vi "Log Results.vi"(8 "Error In":errorcluster, 10 "Warnings":string[](array[string]), 11 "Revert Worker Config":T1={"Job Queue"=refnum, "Job Done Queue"=refnum, "Source Directory"=path "", "Unzip Directory"=path "", "Backsave Directory"=path "", "Output Directory"=path "", "Source File Name"="", "Output Path"="", "LabVIEW Version"=enum."13.0", "Archive Directory"=path ""}) -> (0 "Error Out":errorcluster, 3 "Revert Worker Config":T1={"Job Queue"=refnum, "Job Done Queue"=refnum, "Source Directory"=path "", "Unzip Directory"=path "", "Backsave Directory"=path "", "Output Directory"=path "", "Source File Name"="", "Output Path"="", "LabVIEW Version"=enum."13.0", "Archive Directory"=path ""})   [LabVIEW 2013, in "LVH-Revert.lvlib"]
uses:
  <vilib>/LabVIEW Hacker/Revert/LVH-Revert.lvlib
  <vilib>/LabVIEW Hacker/Revert/Private/Revert Worker Config.ctl
  <vilib>/National Instruments/NI Amazon Web Services (AWS) Toolkit for LabVIEW/SQS/VI Source/AWS SQS Class/AWS_SQS.lvclass
  <vilib>/National Instruments/NI Amazon Web Services (AWS) Toolkit for LabVIEW/AWS Core Lib/VI Source/Canonicals/AWS_Core Canonical Credentials/Canonical Credentials.lvclass
  <vilib>/National Instruments/NI Amazon Web Services (AWS) Toolkit for LabVIEW/AWS Core Lib/VI Source/Canonicals/AWS_Core Canonical Required Parameters/Canonical Required Parameters.lvclass
  <vilib>/National Instruments/NI Amazon Web Services (AWS) Toolkit for LabVIEW/SQS/VI Source/Canonicals/Canonical CreateQueue/Canonical CreateQueue.lvclass
  <vilib>/National Instruments/NI Amazon Web Services (AWS) Toolkit for LabVIEW/SQS/VI Source/Canonicals/Canonical ListQueues/Canonical ListQueues.lvclass
  <vilib>/National Instruments/NI Amazon Web Services (AWS) Toolkit for LabVIEW/SQS/VI Source/Canonicals/Canonical AddPermission/Canonical AddPermission.lvclass
  <vilib>/National Instruments/NI Amazon Web Services (AWS) Toolkit for LabVIEW/SQS/VI Source/Canonicals/Canonical ChangeMessageVisibility/Canonical ChangeMessageVisibility.lvclass
  <vilib>/National Instruments/NI Amazon Web Services (AWS) Toolkit for LabVIEW/SQS/VI Source/Canonicals/Canonical ChangeMessageVisibilityBatch/Canonical ChangeMessageVisibilityBatch.lvclass
  <vilib>/National Instruments/NI Amazon Web Services (AWS) Toolkit for LabVIEW/SQS/VI Source/Canonicals/Canonical DeleteMessage/Canonical DeleteMessage.lvclass
  <vilib>/National Instruments/NI Amazon Web Services (AWS) Toolkit for LabVIEW/SQS/VI Source/Canonicals/Canonical DeleteMessageBatch/Canonical DeleteMessageBatch.lvclass
  <vilib>/National Instruments/NI Amazon Web Services (AWS) Toolkit for LabVIEW/SQS/VI Source/Canonicals/Canonical GetQueueAttributes/Canonical GetQueueAttributes.lvclass
  <vilib>/National Instruments/NI Amazon Web Services (AWS) Toolkit for LabVIEW/SQS/VI Source/Canonicals/Canonical GetQueueUrl/Canonical GetQueueUrl.lvclass
  <vilib>/National Instruments/NI Amazon Web Services (AWS) Toolkit for LabVIEW/SQS/VI Source/Canonicals/Canonical ReceiveMessage/Canonical ReceiveMessage.lvclass
  <vilib>/National Instruments/NI Amazon Web Services (AWS) Toolkit for LabVIEW/SQS/VI Source/Canonicals/Canonical RemovePermission/Canonical RemovePermission.lvclass
  <vilib>/National Instruments/NI Amazon Web Services (AWS) Toolkit for LabVIEW/SQS/VI Source/Canonicals/Canonical SendMessage/Canonical SendMessage.lvclass
  <vilib>/National Instruments/NI Amazon Web Services (AWS) Toolkit for LabVIEW/SQS/VI Source/Canonicals/Canonical SendMessageBatch/Canonical SendMessageBatch.lvclass
  <vilib>/National Instruments/NI Amazon Web Services (AWS) Toolkit for LabVIEW/SQS/VI Source/Canonicals/Canonical SetQueueAttributes/Canonical SetQueueAttributes.lvclass
  <vilib>/LabVIEW Hacker/LVH-Toolbox/Common/Private/Type Defs/LabVIEW Version.ctl
  <vilib>/LabVIEW Hacker/LVH-Toolbox/Common/LVH-Common.lvlib
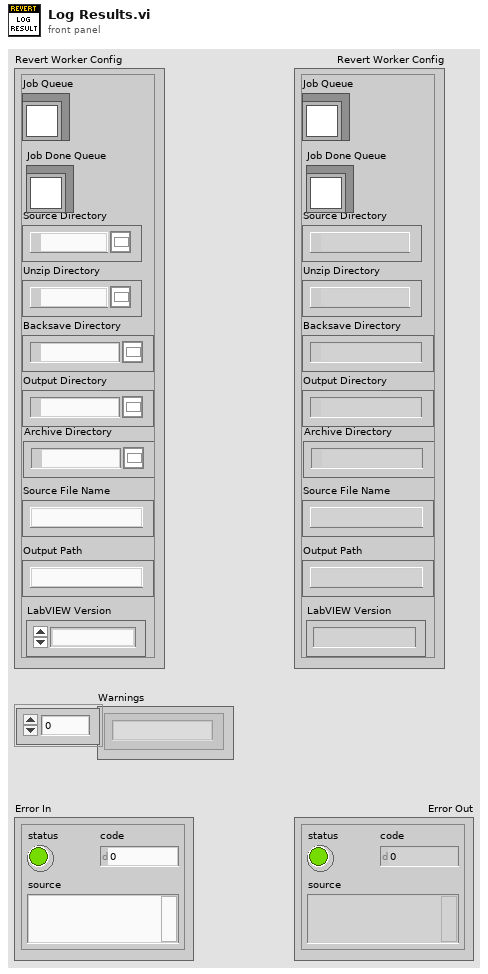
[diagram p1: front panel]
types:
  T1 = typedef "LVH-Revert.lvlib/Revert Worker Config.ctl" = cluster{"Job Queue":refnum<class "AWS_SQS.lvclass">, "Job Done Queue":refnum<class "AWS_SQS.lvclass">, "Source Directory":path, "Unzip Directory":path, "Backsave Directory":path, "Output Directory":path, "Source File Name":string, "Output Path":string, "LabVIEW Version":T2, "Archive Directory":path}
  T2 = typedef "LVH-Toolbox.lvlib/LVH-Common.lvlib/LabVIEW Version.ctl" = enum16{"8.0", "8.2", "8.6", "9.0", "10.0", "11.0", "12.0", "13.0"}
  T3 = enum16{"open", "replace", "create", "open or create", "replace or create", "replace or create with confirmation"}
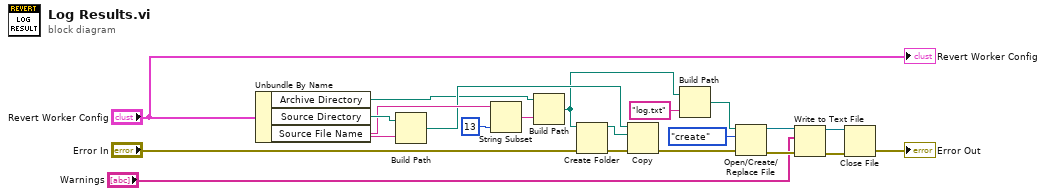
[diagram p0: block diagram]
diagram:
  n1 = Unbundle By Name("Revert Worker Config") -> ("Archive Directory"=w1:path, "Source Directory"=w7:path, "Source File Name"=w6:string)
  n2 = Build Path(base path=w7, name or relative path=w6) -> (appended path=w5:path)
  n3 = String Subset(string=w6, length (rest)=13 ("length (rest)")) -> (substring=w20:string)  [unwired: 1 in]
  n4 = Build Path(base path=w1, name or relative path=w20) -> (appended path=w4:path)
  n5 = Create Folder(path (use dialog)=w4, error in="Error In") -> (created path=w18:path, error out=w19:errorcluster)  [unwired: 1 in, 1 out]
  n6 = Copy(8:w19, 10:w18, 11:w5) -> (0:w17:errorcluster)  [unwired: 2 in, 2 out]
  n7 = Build Path(base path=w4, name or relative path="log.txt") -> (appended path=w15:path)
  n8 = Open/Create/Replace File(file path (use dialog)=w15, error in=w17, operation (0:open)=T3."create") -> (refnum out=w12:refnum<file>, error out=w14:errorcluster)  [unwired: 3 in, 1 out]
  n9 = Write to Text File(file (use dialog)=w12, text="Warnings", error in=w14) -> (refnum out=w9:refnum<file>, error out=w10:errorcluster)  [unwired: 1 in, 1 out]
  n10 = Close File(refnum=w9, error in=w10) -> (error out=→"Error Out":errorcluster)  [unwired: 1 out]
  "Revert Worker Config" <- "Revert Worker Config"
